vi "Valve_Switching_Test.vi"() -> ()   [LabVIEW 2010]
uses:
  labbCAN_Bus_API/labbCAN_Bus_API.lvlib
  labbCAN_Valve_API/labbCAN_Valve_API.lvlib
panel:
  out "Valve count":i32
  out "Available Valves":string[](array[string])
  out "Actual valve position":i32
  out "Valve Position Count":i32
  out "error out":errorcluster caption="Fehler (Ausgang)"
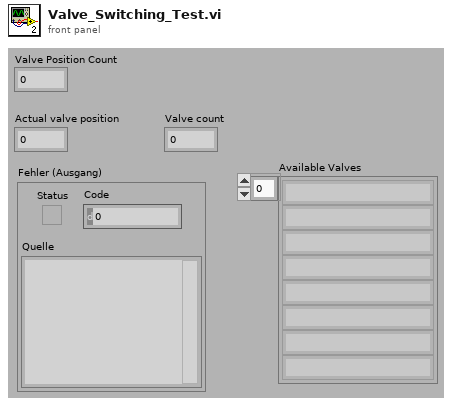
[diagram p1: front panel]
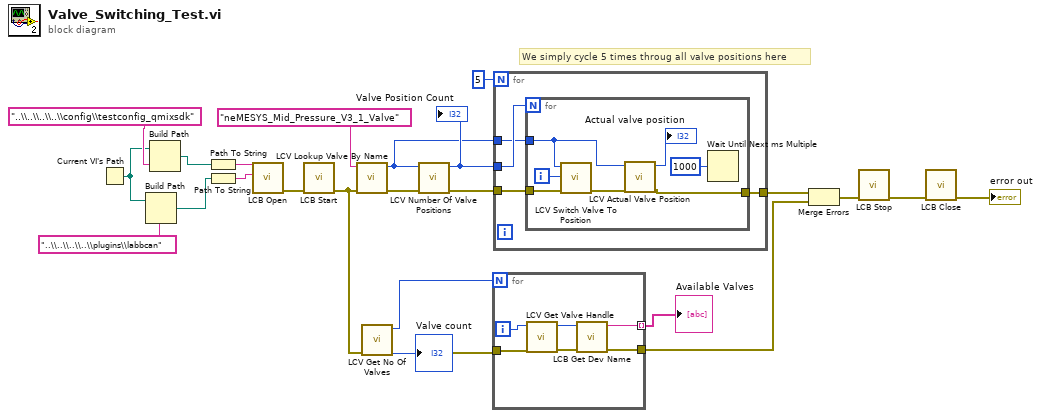
[diagram p0: block diagram]
diagram:
  # "We simply cycle 5 times throug all valve positions here"
  n1 = Current VI's Path() -> (path=w17:path)
  n2 = Build Path(base path=w17, name or relative path="..\\..\\..\\..\\plugins\\labbcan" ("Name oder relativer Pfad")) -> (appended path=w20:path)
  n3 = Build Path(base path=w17, name or relative path="..\\..\\..\\..\\config\\testconfig_qmixsdk" ("Name oder relativer Pfad")) -> (appended path=w16:path)
  n4 = Path To String(path=w16) -> (string=w2:string)
  n5 = Path To String(path=w20) -> (string=w18:string)
  n6 = call "LCB Open.vi"("PluginSearchPath"=w18, "Device Configuration Path"=w2) -> ("error out"=w14:errorcluster)  [unwired: 9 in]
  n7 = call "LCB Start.vi"("error in (no error)"=w14) -> ("error out"=w8:errorcluster)  [unwired: 10 in]
  n8 = call "LCV Lookup Valve By Name.vi"("error in (no error)"=w8, "Valve Name"="neMESYS_Mid_Pressure_V3_1_Valve") -> ("error out"=w13:errorcluster, "Valve handle"=w9:i64)  [unwired: 8 in]
  n9 = call "LCV Get No Of Valves.vi"("error in (no error)"=w8) -> ("error out"=w6:errorcluster, "Valve count"=w7:i32)  [unwired: 9 in]
  "Valve count" <- w7
  n10 = call "LCV Number Of Valve Positions.vi"("error in (no error)"=w13, "Valve Handle"=w9) -> ("error out"=w10:errorcluster, "Valve Position Count"=w11:i32)  [unwired: 8 in]
  "Valve Position Count" <- w11
  n11 = for {
    N: w7 -> [_]
    tunnel: w6 -> [w29]
    tunnel: [w25] -> w3
    tunnel: [w24] -> w1 mode=indexing
    i -> [w28]
    n12 = call "LCV Get Valve Handle.vi"("error in (no error)"=w29, "Valve Index"=w28) -> ("error out"=w27:errorcluster, "Valve handle"=w26:i64)  [unwired: 8 in]
    n13 = call "LCB Get Dev Name.vi"("error in (no error)"=w27, "Device Handle"=w26) -> ("error out"=w25:errorcluster, "Device Name"=w24:string)  [unwired: 8 in]
  }
  "Available Valves" <- w1
  n14 = for {
    N: 5 -> [_]
    tunnel: w11 -> [w33]
    tunnel: w10 -> [w32]
    tunnel: w9 -> [w31]
    tunnel: [w30] -> w5
    n15 = for {
      N: w33 -> [_]
      tunnel: w32 -> [w40]
      tunnel: w31 -> [w37]
      tunnel: [w35] -> w30
      i -> [w39]
      n16 = call "LCV Switch Valve To Position.vi"("error in (no error)"=w40, "Logical Valve Position"=w39, "Valve Handle"=w37) -> ("error out"=w38:errorcluster)  [unwired: 8 in]
      n17 = call "LCV Actual Valve Position.vi"("error in (no error)"=w38, "Valve Handle"=w37) -> ("error out"=w35:errorcluster, "Actual valve position"=→"Actual valve position":i32)  [unwired: 8 in]
      n18 = Wait Until Next ms Multiple(millisecond multiple=u32 1000 ("Vielfache von ms")) -> ()  [unwired: 1 out]
    }
  }
  n19 = Merge Errors(w5, w3) -> (w4:errorcluster)
  n20 = call "LCB Stop.vi"("error in (no error)"=w4) -> ("error out"=w22:errorcluster)  [unwired: 10 in]
  n21 = call "LCB Close.vi"("error in (no error)"=w22) -> ("error out"=→"error out":errorcluster)  [unwired: 10 in]
